vi "Status 2 Write.vi"(4 "error in (no error)":errorcluster, 5 "Value":cluster{"BG":u32, "FG":u32}, 6 "Container State":T2, 7 "Display State In":T1={"State 1"={"BG"=0, "FG"=0}, "State 0"={"BG"=0, "FG"=0}, "State 2"={"BG"=0, "FG"=0}, "State 3"={"BG"=0, "FG"=0}, "Shortcut Menu"=enum."Do left-click popup"}) -> (0 "error out":errorcluster, 3 "Display State Out":T1={"State 1"={"BG"=0, "FG"=0}, "State 0"={"BG"=0, "FG"=0}, "State 2"={"BG"=0, "FG"=0}, "State 3"={"BG"=0, "FG"=0}, "Shortcut Menu"=enum."Do left-click popup"})   [LabVIEW 2011, in "Led.xctl"]
uses:
  Led.xctl
  <vilib>/_xctls/Container State.ctl
  State.ctl
  <vilib>/_xctls/XControlSupport.lvlib
panel:
  # "Replace the Value Control below with a Control of desired type.\nDo not remove this Control or the others from the connector pane.\nDo not change the connector pane pattern.\nThe Value control should always be the third terminal from top on the input side in the connector pane."
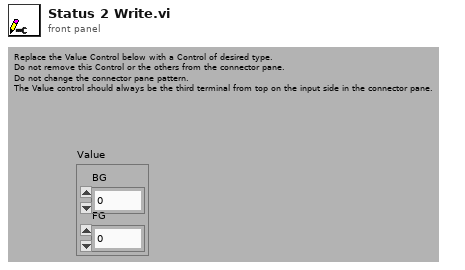
[diagram p1: front panel]
types:
  T1 = typedef "Led.xctl/State.ctl" = cluster{"State 1":cluster{"BG":u32, "FG":u32}, "State 0":cluster{"BG":u32, "FG":u32}, "State 2":cluster{"BG":u32, "FG":u32}, "State 3":cluster{"BG":u32, "FG":u32}, "Shortcut Menu":enum16{"Treat normally", "Do left-click popup"}}
  T2 = typedef "XControlSupport.lvlib/Container State.ctl" = cluster{"Indicator?":bool, "Run Mode?":bool, " Refnum":refnum<vi>}
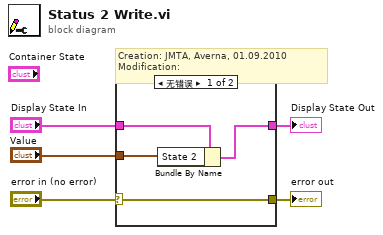
[diagram p0: block diagram]
diagram:
  # "Creation: JMTA, Averna, 01.09.2010 \nModification:"
  n1 = case shown="无错误" "error in (no error)" {
    selector: "error in (no error)" -> [w9 w10]
    tunnel: "Display State In" -> [w7 w11]
    tunnel: [w9 w10] -> w3
    tunnel: [w6 w11] -> w1
    tunnel: "Value" -> [w8 _]
    frame No Error {
      n2 = Bundle By Name(cluster=w7, "State 2"=w8) -> (w6:T1)
    }
    frame Error {
    }
  }
  "error out" <- w3
  "Display State Out" <- w1
